vi "Create-Destroy.vi"(7 "Address":string, 8 "Error In":errorcluster) -> (0 "Error Out":errorcluster)   [LabVIEW 2018, in "Tests.lvlib" / "Known Hosts.lvlib"]
uses:
  Known Hosts.lvlib
  <vilib>/addons/_JKI Toolkits/Caraya/classes/Test/Test.lvclass
  <vilib>/addons/_JKI Toolkits/Caraya/classes/Assert/Assert.lvclass
  src/Toolkit/Known Hosts/Known Hosts.lvclass
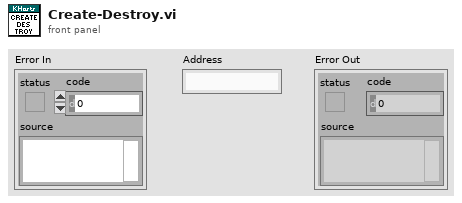
[diagram p1: front panel]
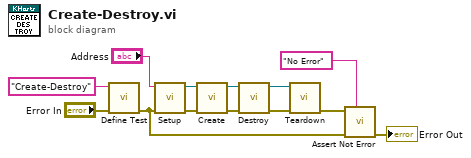
[diagram p0: block diagram]
diagram:
  n1 = call <vilib>:"Define Test.vi"("error in (no error)"="Error In", "Label (VI Title)"="Create-Destroy") -> ("error out"=w4:errorcluster)  [unwired: 9 in]
  n2 = call "Setup.vi"("Error In"=w4, "Address In"="Address") -> ("Error Out"=w5:errorcluster, "Sesssion"=w2:refnum<class "Session.lvclass">)  [unwired: 7 in, 1 out]
  n3 = call "Create.vi"("Error In"=w5, "Session"=w2) -> ("Error Out"=w7:errorcluster, "Known Hosts"=w8:refnum<class "Known Hosts.lvclass">)  [unwired: 8 in]
  n4 = call "Destroy.vi"("Error In"=w7, "KnownHosts"=w8) -> ("Error Out"=w6:errorcluster, "Session"=w1:refnum<class "Session.lvclass">)  [unwired: 8 in]
  n5 = call "Teardown.vi"("Error In"=w6, "Session"=w1) -> ("Error Out"=w11:errorcluster)  [unwired: 9 in]
  n6 = call <vilib>:"Assert Not Error.vi"("Label"="No Error", "error in (no error)"=w4, "Not Error?"=w11) -> ("error out"=→"Error Out":errorcluster)  [unwired: 8 in]
